vi "FipsAdjacent.vi"() -> (11 "Fips":i32[](array[numeric]))   [LabVIEW 2017] (continued)
 County, WI\"\t55119\n\"Manitowoc County, WI\"\t55071\t\"Manistee County, MI\"\t26101\n\"Manitowoc County, WI\"\t55071\t\"Mason County, MI\"\t26105\n\"Manitowoc County, WI\"\t55071\t\"Brown County, WI\"\t55009\n\"Manitowoc County, WI\"\t55071\t\"Calumet County, WI\"\t55015\n\"Manitowoc County, WI\"\t55071\t\"Kewaunee County, WI\"\t55061\n\"Manitowoc County, WI\"\t55071\t\"Manitowoc County, WI\"\t55071\n\"Manitowoc County, WI\"\t55071\t\"Sheboygan County, WI\"\t55117\n\"Marathon County, WI\"\t55073\t\"Clark County, WI\"\t55019\n\"Marathon County, WI\"\t55073\t\"Langlade County, WI\"\t55067\n\"Marathon County, WI\"\t55073\t\"Lincoln County, WI\"\t55069\n\"Marathon County, WI\"\t55073\t\"Marathon County, WI\"\t55073\n\"Marathon County, WI\"\t55073\t\"Portage County, WI\"\t55097\n\"Marathon County, WI\"\t55073\t\"Shawano County, WI\"\t55115\n\"Marathon County, WI\"\t55073\t\"Taylor County, WI\"\t55119\n\"Marathon County, WI\"\t55073\t\"Waupaca County, WI\"\t55135\n\"Marathon County, WI\"\t55073\t\"Wood County, WI\"\t55141\n\"Marinette County, WI\"\t55075\t\"Dickinson County, MI\"\t26043\n\"Marinette County, WI\"\t55075\t\"Menominee County, MI\"\t26109\n\"Marinette County, WI\"\t55075\t\"Door County, WI\"\t55029\n\"Marinette County, WI\"\t55075\t\"Florence County, WI\"\t55037\n\"Marinette County, WI\"\t55075\t\"Forest County, WI\"\t55041\n\"Marinette County, WI\"\t55075\t\"Marinette County, WI\"\t55075\n\"Marinette County, WI\"\t55075\t\"Oconto County, WI\"\t55083\n\"Marquette County, WI\"\t55077\t\"Adams County, WI\"\t55001\n\"Marquette County, WI\"\t55077\t\"Columbia County, WI\"\t55021\n\"Marquette County, WI\"\t55077\t\"Green Lake County, WI\"\t55047\n\"Marquette County, WI\"\t55077\t\"Marquette County, WI\"\t55077\n\"Marquette County, WI\"\t55077\t\"Waushara County, WI\"\t55137\n\"Menominee County, WI\"\t55078\t\"Langlade County, WI\"\t55067\n\"Menominee County, WI\"\t55078\t\"Menominee County, WI\"\t55078\n\"Menominee County, WI\"\t55078\t\"Oconto County, WI\"\t55083\n\"Menominee County, WI\"\t55078\t\"Shawano County, WI\"\t55115\n\"Milwaukee County, WI\"\t55079\t\"Muskegon County, MI\"\t26121\n\"Milwaukee County, WI\"\t55079\t\"Ottawa County, MI\"\t26139\n\"Milwaukee County, WI\"\t55079\t\"Milwaukee County, WI\"\t55079\n\"Milwaukee County, WI\"\t55079\t\"Ozaukee County, WI\"\t55089\n\"Milwaukee County, WI\"\t55079\t\"Racine County, WI\"\t55101\n\"Milwaukee County, WI\"\t55079\t\"Washington County, WI\"\t55131\n\"Milwaukee County, WI\"\t55079\t\"Waukesha County, WI\"\t55133\n\"Monroe County, WI\"\t55081\t\"Jackson County, WI\"\t55053\n\"Monroe County, WI\"\t55081\t\"Juneau County, WI\"\t55057\n\"Monroe County, WI\"\t55081\t\"La Crosse County, WI\"\t55063\n\"Monroe County, WI\"\t55081\t\"Monroe County, WI\"\t55081\n\"Monroe County, WI\"\t55081\t\"Vernon County, WI\"\t55123\n\"Oconto County, WI\"\t55083\t\"Brown County, WI\"\t55009\n\"Oconto County, WI\"\t55083\t\"Door County, WI\"\t55029\n\"Oconto County, WI\"\t55083\t\"Forest County, WI\"\t55041\n\"Oconto County, WI\"\t55083\t\"Langlade County, WI\"\t55067\n\"Oconto County, WI\"\t55083\t\"Marinette County, WI\"\t55075\n\"Oconto County, WI\"\t55083\t\"Menominee County, WI\"\t55078\n\"Oconto County, WI\"\t55083\t\"Oconto County, WI\"\t55083\n\"Oconto County, WI\"\t55083\t\"Shawano County, WI\"\t55115\n\"Oneida County, WI\"\t55085\t\"Forest County, WI\"\t55041\n\"Oneida County, WI\"\t55085\t\"Langlade County, WI\"\t55067\n\"Oneida County, WI\"\t55085\t\"Lincoln County, WI\"\t55069\n\"Oneida County, WI\"\t55085\t\"Oneida County, WI\"\t55085\n\"Oneida County, WI\"\t55085\t\"Price County, WI\"\t55099\n\"Oneida County, WI\"\t55085\t\"Vilas County, WI\"\t55125\n\"Outagamie County, WI\"\t55087\t\"Brown County, WI\"\t55009\n\"Outagamie County, WI\"\t55087\t\"Calumet County, WI\"\t55015\n\"Outagamie County, WI\"\t55087\t\"Outagamie County, WI\"\t55087\n\"Outagamie County, WI\"\t55087\t\"Shawano County, WI\"\t55115\n\"Outagamie County, WI\"\t55087\t\"Waupaca County, WI\"\t55135\n\"Outagamie County, WI\"\t55087\t\"Winnebago County, WI\"\t55139\n\"Ozaukee County, WI\"\t55089\t\"Muskegon County, MI\"\t26121\n\"Ozaukee County, WI\"\t55089\t\"Oceana County, MI\"\t26127\n\"Ozaukee County, WI\"\t55089\t\"Milwaukee County, WI\"\t55079\n\"Ozaukee County, WI\"\t55089\t\"Ozaukee County, WI\"\t55089\n\"Ozaukee County, WI\"\t55089\t\"Sheboygan County, WI\"\t55117\n\"Ozaukee County, WI\"\t55089\t\"Washington County, WI\"\t55131\n\"Ozaukee County, WI\"\t55089\t\"Waukesha County, WI\"\t55133\n\"Pepin County, WI\"\t55091\t\"Goodhue County, MN\"\t27049\n\"Pepin County, WI\"\t55091\t\"Wabasha County, MN\"\t27157\n\"Pepin County, WI\"\t55091\t\"Buffalo County, WI\"\t55011\n\"Pepin County, WI\"\t55091\t\"Dunn County, WI\"\t55033\n\"Pepin County, WI\"\t55091\t\"Eau Claire County, WI\"\t55035\n\"Pepin County, WI\"\t55091\t\"Pepin County, WI\"\t55091\n\"Pepin County, WI\"\t55091\t\"Pierce County, WI\"\t55093\n\"Pierce County, WI\"\t55093\t\"Dakota County, MN\"\t27037\n\"Pierce County, WI\"\t55093\t\"Goodhue County, MN\"\t27049\n\"Pierce County, WI\"\t55093\t\"Washington County, MN\"\t27163\n\"Pierce County, WI\"\t55093\t\"Dunn County, WI\"\t55033\n\"Pierce County, WI\"\t55093\t\"Pepin County, WI\"\t55091\n\"Pierce County, WI\"\t55093\t\"Pierce County, WI\"\t55093\n\"Pierce County, WI\"\t55093\t\"St. Croix County, WI\"\t55109\n\"Polk County, WI\"\t55095\t\"Chisago County, MN\"\t27025\n\"Polk County, WI\"\t55095\t\"Washington County, MN\"\t27163\n\"Polk County, WI\"\t55095\t\"Barron County, WI\"\t55005\n\"Polk County, WI\"\t55095\t\"Burnett County, WI\"\t55013\n\"Polk County, WI\"\t55095\t\"Dunn County, WI\"\t55033\n\"Polk County, WI\"\t55095\t\"Polk County, WI\"\t55095\n\"Polk County, WI\"\t55095\t\"St. Croix County, WI\"\t55109\n\"Portage County, WI\"\t55097\t\"Adams County, WI\"\t55001\n\"Portage County, WI\"\t55097\t\"Marathon County, WI\"\t55073\n\"Portage County, WI\"\t55097\t\"Portage County, WI\"\t55097\n\"Portage County, WI\"\t55097\t\"Shawano County, WI\"\t55115\n\"Portage County, WI\"\t55097\t\"Waupaca County, WI\"\t55135\n\"Portage County, WI\"\t55097\t\"Waushara County, WI\"\t55137\n\"Portage County, WI\"\t55097\t\"Wood County, WI\"\t55141\n\"Price County, WI\"\t55099\t\"Ashland County, WI\"\t55003\n\"Price County, WI\"\t55099\t\"Iron County, WI\"\t55051\n\"Price County, WI\"\t55099\t\"Lincoln County, WI\"\t55069\n\"Price County, WI\"\t55099\t\"Oneida County, WI\"\t55085\n\"Price County, WI\"\t55099\t\"Price County, WI\"\t55099\n\"Price County, WI\"\t55099\t\"Rusk County, WI\"\t55107\n\"Price County, WI\"\t55099\t\"Sawyer County, WI\"\t55113\n\"Price County, WI\"\t55099\t\"Taylor County, WI\"\t55119\n\"Price County, WI\"\t55099\t\"Vilas County, WI\"\t55125\n\"Racine County, WI\"\t55101\t\"Allegan County, MI\"\t26005\n\"Racine County, WI\"\t55101\t\"Ottawa County, MI\"\t26139\n\"Racine County, WI\"\t55101\t\"Kenosha County, WI\"\t55059\n\"Racine County, WI\"\t55101\t\"Milwaukee County, WI\"\t55079\n\"Racine County, WI\"\t55101\t\"Racine County, WI\"\t55101\n\"Racine County, WI\"\t55101\t\"Walworth County, WI\"\t55127\n\"Racine County, WI\"\t55101\t\"Waukesha County, WI\"\t55133\n\"Richland County, WI\"\t55103\t\"Crawford County, WI\"\t55023\n\"Richland County, WI\"\t55103\t\"Grant County, WI\"\t55043\n\"Richland County, WI\"\t55103\t\"Iowa County, WI\"\t55049\n\"Richland County, WI\"\t55103\t\"Richland County, WI\"\t55103\n\"Richland County, WI\"\t55103\t\"Sauk County, WI\"\t55111\n\"Richland County, WI\"\t55103\t\"Vernon County, WI\"\t55123\n\"Rock County, WI\"\t55105\t\"Boone County, IL\"\t17007\n\"Rock County, WI\"\t55105\t\"Winnebago County, IL\"\t17201\n\"Rock County, WI\"\t55105\t\"Dane County, WI\"\t55025\n\"Rock County, WI\"\t55105\t\"Green County, WI\"\t55045\n\"Rock County, WI\"\t55105\t\"Jefferson County, WI\"\t55055\n\"Rock County, WI\"\t55105\t\"Rock County, WI\"\t55105\n\"Rock County, WI\"\t55105\t\"Walworth County, WI\"\t55127\n\"Rusk County, WI\"\t55107\t\"Barron County, WI\"\t55005\n\"Rusk County, WI\"\t55107\t\"Chippewa County, WI\"\t55017\n\"Rusk County, WI\"\t55107\t\"Price County, WI\"\t55099\n\"Rusk County, WI\"\t55107\t\"Rusk County, WI\"\t55107\n\"Rusk County, WI\"\t55107\t\"Sawyer County, WI\"\t55113\n\"Rusk County, WI\"\t55107\t\"Taylor County, WI\"\t55119\n\"Rusk County, WI\"\t55107\t\"Washburn County, WI\"\t55129\n\"St. Croix County, WI\"\t55109\t\"Washington County, MN\"\t27163\n\"St. Croix County, WI\"\t55109\t\"Barron County, WI\"\t55005\n\"St. Croix County, WI\"\t55109\t\"Dunn County, WI\"\t55033\n\"St. Croix County, WI\"\t55109\t\"Pierce County, WI\"\t55093\n\"St. Croix County, WI\"\t55109\t\"Polk County, WI\"\t55095\n\"St. Croix County, WI\"\t55109\t\"St. Croix County, WI\"\t55109\n\"Sauk County, WI\"\t55111\t\"Adams County, WI\"\t55001\n\"Sauk County, WI\"\t55111\t\"Columbia County, WI\"\t55021\n\"Sauk County, WI\"\t55111\t\"Dane County, WI\"\t55025\n\"Sauk County, WI\"\t55111\t\"Iowa County, WI\"\t55049\n\"Sauk County, WI\"\t55111\t\"Juneau County, WI\"\t55057\n\"Sauk County, WI\"\t55111\t\"Richland County, WI\"\t55103\n\"Sauk County, WI\"\t55111\t\"Sauk County, WI\"\t55111\n\"Sauk County, WI\"\t55111\t\"Vernon County, WI\"\t55123\n\"Sawyer County, WI\"\t55113\t\"Ashland County, WI\"\t55003\n\"Sawyer County, WI\"\t55113\t\"Barron County, WI\"\t55005\n\"Sawyer County, WI\"\t55113\t\"Bayfield County, WI\"\t55007\n\"Sawyer County, WI\"\t55113\t\"Douglas County, WI\"\t55031\n\"Sawyer County, WI\"\t55113\t\"Price County, WI\"\t55099\n\"Sawyer County, WI\"\t55113\t\"Rusk County, WI\"\t55107\n\"Sawyer County, WI\"\t55113\t\"Sawyer County, WI\"\t55113\n\"Sawyer County, WI\"\t55113\t\"Washburn County, WI\"\t55129\n\"Shawano County, WI\"\t55115\t\"Brown County, WI\"\t55009\n\"Shawano County, WI\"\t55115\t\"Langlade County, WI\"\t55067\n\"Shawano County, WI\"\t55115\t\"Marathon County, WI\"\t55073\n\"Shawano County, WI\"\t55115\t\"Menominee County, WI\"\t55078\n\"Shawano County, WI\"\t55115\t\"Oconto County, WI\"\t55083\n\"Shawano County, WI\"\t55115\t\"Outagamie County, WI\"\t55087\n\"Shawano County, WI\"\t55115\t\"Portage County, WI\"\t55097\n\"Shawano County, WI\"\t55115\t\"Shawano County, WI\"\t55115\n\"Shawano County, WI\"\t55115\t\"Waupaca County, WI\"\t55135\n\"Sheboygan County, WI\"\t55117\t\"Mason County, MI\"\t26105\n\"Sheboygan County, WI\"\t55117\t\"Oceana County, MI\"\t26127\n\"Sheboygan County, WI\"\t55117\t\"Calumet County, WI\"\t55015\n\"Sheboygan County, WI\"\t55117\t\"Fond du Lac County, WI\"\t55039\n\"Sheboygan County, WI\"\t55117\t\"Manitowoc County, WI\"\t55071\n\"Sheboygan County, WI\"\t55117\t\"Ozaukee County, WI\"\t55089\n\"Sheboygan County, WI\"\t55117\t\"Sheboygan County, WI\"\t55117\n\"Sheboygan County, WI\"\t55117\t\"Washington County, WI\"\t55131\n\"Taylor County, WI\"\t55119\t\"Chippewa County, WI\"\t55017\n\"Taylor County, WI\"\t55119\t\"Clark County, WI\"\t55019\n\"Taylor County, WI\"\t55119\t\"Lincoln County, WI\"\t55069\n\"Taylor County, WI\"\t55119\t\"Marathon County, WI\"\t55073\n\"Taylor County, WI\"\t55119\t\"Price County, WI\"\t55099\n\"Taylor County, WI\"\t55119\t\"Rusk County, WI\"\t55107\n\"Taylor County, WI\"\t55119\t\"Taylor County, WI\"\t55119\n\"Trempealeau County, WI\"\t55121\t\"Winona County, MN\"\t27169\n\"Trempealeau County, WI\"\t55121\t\"Buffalo County, WI\"\t55011\n\"Trempealeau County, WI\"\t55121\t\"Eau Claire County, WI\"\t55035\n\"Trempealeau County, WI\"\t55121\t\"Jackson County, WI\"\t55053\n\"Trempealeau County, WI\"\t55121\t\"La Crosse County, WI\"\t55063\n\"Trempealeau County, WI\"\t55121\t\"Trempealeau County, WI\"\t55121\n\"Vernon County, WI\"\t55123\t\"Allamakee County, IA\"\t19005\n\"Vernon County, WI\"\t55123\t\"Houston County, MN\"\t27055\n\"Vernon County, WI\"\t55123\t\"Crawford County, WI\"\t55023\n\"Vernon County, WI\"\t55123\t\"Juneau County, WI\"\t55057\n\"Vernon County, WI\"\t55123\t\"La Crosse County, WI\"\t55063\n\"Vernon County, WI\"\t55123\t\"Monroe County, WI\"\t55081\n\"Vernon County, WI\"\t55123\t\"Richland County, WI\"\t55103\n\"Vernon County, WI\"\t55123\t\"Sauk County, WI\"\t55111\n\"Vernon County, WI\"\t55123\t\"Vernon County, WI\"\t55123\n\"Vilas County, WI\"\t55125\t\"Gogebic County, MI\"\t26053\n\"Vilas County, WI\"\t55125\t\"Iron County, MI\"\t26071\n\"Vilas County, WI\"\t55125\t\"Forest County, WI\"\t55041\n\"Vilas County, WI\"\t55125\t\"Iron County, WI\"\t55051\n\"Vilas County, WI\"\t55125\t\"Oneida County, WI\"\t55085\n\"Vilas County, WI\"\t55125\t\"Price County, WI\"\t55099\n\"Vilas County, WI\"\t55125\t\"Vilas County, WI\"\t55125\n\"Walworth County, WI\"\t55127\t\"Boone County, IL\"\t17007\n\"Walworth County, WI\"\t55127\t\"McHenry County, IL\"\t17111\n\"Walworth County, WI\"\t55127\t\"Jefferson County, WI\"\t55055\n\"Walworth County, WI\"\t55127\t\"Kenosha County, WI\"\t55059\n\"Walworth County, WI\"\t55127\t\"Racine County, WI\"\t55101\n\"Walworth County, WI\"\t55127\t\"Rock County, WI\"\t55105\n\"Walworth County, WI\"\t55127\t\"Walworth County, WI\"\t55127\n\"Walworth County, WI\"\t55127\t\"Waukesha County, WI\"\t55133\n\"Washburn County, WI\"\t55129\t\"Barron County, WI\"\t55005\n\"Washburn County, WI\"\t55129\t\"Bayfield County, WI\"\t55007\n\"Washburn County, WI\"\t55129\t\"Burnett County, WI\"\t55013\n\"Washburn County, WI\"\t55129\t\"Douglas County, WI\"\t55031\n\"Washburn County, WI\"\t55129\t\"Rusk County, WI\"\t55107\n\"Washburn County, WI\"\t55129\t\"Sawyer County, WI\"\t55113\n\"Washburn County, WI\"\t55129\t\"Washburn County, WI\"\t55129\n\"Washington County, WI\"\t55131\t\"Dodge County, WI\"\t55027\n\"Washington County, WI\"\t55131\t\"Fond du Lac County, WI\"\t55039\n\"Washington County, WI\"\t55131\t\"Milwaukee County, WI\"\t55079\n\"Washington County, WI\"\t55131\t\"Ozaukee County, WI\"\t55089\n\"Washington County, WI\"\t55131\t\"Sheboygan County, WI\"\t55117\n\"Washington County, WI\"\t55131\t\"Washington County, WI\"\t55131\n\"Washington County, WI\"\t55131\t\"Waukesha County, WI\"\t55133\n\"Waukesha County, WI\"\t55133\t\"Dodge County, WI\"\t55027\n\"Waukesha County, WI\"\t55133\t\"Jefferson County, WI\"\t55055\n\"Waukesha County, WI\"\t55133\t\"Milwaukee County, WI\"\t55079\n\"Waukesha County, WI\"\t55133\t\"Ozaukee County, WI\"\t55089\n\"Waukesha County, WI\"\t55133\t\"Racine County, WI\"\t55101\n\"Waukesha County, WI\"\t55133\t\"Walworth County, WI\"\t55127\n\"Waukesha County, WI\"\t55133\t\"Washington County, WI\"\t55131\n\"Waukesha County, WI\"\t55133\t\"Waukesha County, WI\"\t55133\n\"Waupaca County, WI\"\t55135\t\"Marathon County, WI\"\t55073\n\"Waupaca County, WI\"\t55135\t\"Outagamie County, WI\"\t55087\n\"Waupaca County, WI\"\t55135\t\"Portage County, WI\"\t55097\n\"Waupaca County, WI\"\t55135\t\"Shawano County, WI\"\t55115\n\"Waupaca County, WI\"\t55135\t\"Waupaca County, WI\"\t55135\n\"Waupaca County, WI\"\t55135\t\"Waushara County, WI\"\t55137\n\"Waupaca County, WI\"\t55135\t\"Winnebago County, WI\"\t55139\n\"Waushara County, WI\"\t55137\t\"Adams County, WI\"\t55001\n\"Waushara County, WI\"\t55137\t\"Green Lake County, WI\"\t55047\n\"Waushara County, WI\"\t55137\t\"Marquette County, WI\"\t55077\n\"Waushara County, WI\"\t55137\t\"Portage County, WI\"\t55097\n\"Waushara County, WI\"\t55137\t\"Waupaca County, WI\"\t55135\n\"Waushara County, WI\"\t55137\t\"Waushara County, WI\"\t55137\n\"Waushara County, WI\"\t55137\t\"Winnebago County, WI\"\t55139\n\"Winnebago County, WI\"\t55139\t\"Calumet County, WI\"\t55015\n\"Winnebago County, WI\"\t55139\t\"Fond du Lac County, WI\"\t55039\n\"Winnebago County, WI\"\t55139\t\"Green Lake County, WI\"\t55047\n\"Winnebago County, WI\"\t55139\t\"Outagamie County, WI\"\t55087\n\"Winnebago County, WI\"\t55139\t\"Waupaca County, WI\"\t55135\n\"Winnebago County, WI\"\t55139\t\"Waushara County, WI\"\t55137\n\"Winnebago County, WI\"\t55139\t\"Winnebago County, WI\"\t55139\n\"Wood County, WI\"\t55141\t\"Adams County, WI\"\t55001\n\"Wood County, WI\"\t55141\t\"Clark County, WI\"\t55019\n\"Wood County, WI\"\t55141\t\"Jackson County, WI\"\t55053\n\"Wood County, WI\"\t55141\t\"Juneau County, WI\"\t55057\n\"Wood County, WI\"\t55141\t\"Marathon County, WI\"\t55073\n\"Wood County, WI\"\t55141\t\"Portage County, WI\"\t55097\n\"Wood County, WI\"\t55141\t\"Wood County, WI\"\t55141\n\"Albany County, WY\"\t56001\t\"Jackson County, CO\"\t08057\n\"Albany County, WY\"\t56001\t\"Larimer County, CO\"\t08069\n\"Albany County, WY\"\t56001\t\"Albany County, WY\"\t56001\n\"Albany County, WY\"\t56001\t\"Carbon County, WY\"\t56007\n\"Albany County, WY\"\t56001\t\"Converse County, WY\"\t56009\n\"Albany County, WY\"\t56001\t\"Laramie County, WY\"\t56021\n\"Albany County, WY\"\t56001\t\"Platte County, WY\"\t56031\n\"Big Horn County, WY\"\t56003\t\"Big Horn County, MT\"\t30003\n\"Big Horn County, WY\"\t56003\t\"Carbon County, MT\"\t30009\n\"Big Horn County, WY\"\t56003\t\"Big Horn County, WY\"\t56003\n\"Big Horn County, WY\"\t56003\t\"Johnson County, WY\"\t56019\n\"Big Horn County, WY\"\t56003\t\"Park County, WY\"\t56029\n\"Big Horn County, WY\"\t56003\t\"Sheridan County, WY\"\t56033\n\"Big Horn County, WY\"\t56003\t\"Washakie County, WY\"\t56043\n\"Campbell County, WY\"\t56005\t\"Powder River County, MT\"\t30075\n\"Campbell County, WY\"\t56005\t\"Campbell County, WY\"\t56005\n\"Campbell County, WY\"\t56005\t\"Converse County, WY\"\t56009\n\"Campbell County, WY\"\t56005\t\"Crook County, WY\"\t56011\n\"Campbell County, WY\"\t56005\t\"Johnson County, WY\"\t56019\n\"Campbell County, WY\"\t56005\t\"Sheridan County, WY\"\t56033\n\"Campbell County, WY\"\t56005\t\"Weston County, WY\"\t56045\n\"Carbon County, WY\"\t56007\t\"Jackson County, CO\"\t08057\n\"Carbon County, WY\"\t56007\t\"Moffat County, CO\"\t08081\n\"Carbon County, WY\"\t56007\t\"Routt County, CO\"\t08107\n\"Carbon County, WY\"\t56007\t\"Albany County, WY\"\t56001\n\"Carbon County, WY\"\t56007\t\"Carbon County, WY\"\t56007\n\"Carbon County, WY\"\t56007\t\"Converse County, WY\"\t56009\n\"Carbon County, WY\"\t56007\t\"Fremont County, WY\"\t56013\n\"Carbon County, WY\"\t56007\t\"Natrona County, WY\"\t56025\n\"Carbon County, WY\"\t56007\t\"Sweetwater County, WY\"\t56037\n\"Converse County, WY\"\t56009\t\"Albany County, WY\"\t56001\n\"Converse County, WY\"\t56009\t\"Campbell County, WY\"\t56005\n\"Converse County, WY\"\t56009\t\"Carbon County, WY\"\t56007\n\"Converse County, WY\"\t56009\t\"Converse County, WY\"\t56009\n\"Converse County, WY\"\t56009\t\"Johnson County, WY\"\t56019\n\"Converse County, WY\"\t56009\t\"Natrona County, WY\"\t56025\n\"Converse County, WY\"\t56009\t\"Niobrara County, WY\"\t56027\n\"Converse County, WY\"\t56009\t\"Platte County, WY\"\t56031\n\"Converse County, WY\"\t56009\t\"Weston County, WY\"\t56045\n\"Crook County, WY\"\t56011\t\"Carter County, MT\"\t30011\n\"Crook County, WY\"\t56011\t\"Powder River County, MT\"\t30075\n\"Crook County, WY\"\t56011\t\"Butte County, SD\"\t46019\n\"Crook County, WY\"\t56011\t\"Lawrence County, SD\"\t46081\n\"Crook County, WY\"\t56011\t\"Campbell County, WY\"\t56005\n\"Crook County, WY\"\t56011\t\"Crook County, WY\"\t56011\n\"Crook County, WY\"\t56011\t\"Weston County, WY\"\t56045\n\"Fremont County, WY\"\t56013\t\"Carbon County, WY\"\t56007\n\"Fremont County, WY\"\t56013\t\"Fremont County, WY\"\t56013\n\"Fremont County, WY\"\t56013\t\"Hot Springs County, WY\"\t56017\n\"Fremont County, WY\"\t56013\t\"Natrona County, WY\"\t56025\n\"Fremont County, WY\"\t56013\t\"Park County, WY\"\t56029\n\"Fremont County, WY\"\t56013\t\"Sublette County, WY\"\t56035\n\"Fremont County, WY\"\t56013\t\"Sweetwater County, WY\"\t56037\n\"Fremont County, WY\"\t56013\t\"Teton County, WY\"\t56039\n\"Fremont County, WY\"\t56013\t\"Washakie County, WY\"\t56043\n\"Goshen County, WY\"\t56015\t\"Banner County, NE\"\t31007\n\"Goshen County, WY\"\t56015\t\"Scotts Bluff County, NE\"\t31157\n\"Goshen County, WY\"\t56015\t\"Sioux County, NE\"\t31165\n\"Goshen County, WY\"\t56015\t\"Goshen County, WY\"\t56015\n\"Goshen County, WY\"\t56015\t\"Laramie County, WY\"\t56021\n\"Goshen County, WY\"\t56015\t\"Niobrara County, WY\"\t56027\n\"Goshen County, WY\"\t56015\t\"Platte County, WY\"\t56031\n\"Hot Springs County, WY\"\t56017\t\"Fremont County, WY\"\t56013\n\"Hot Springs County, WY\"\t56017\t\"Hot Springs County, WY\"\t56017\n\"Hot Springs County, WY\"\t56017\t\"Park County, WY\"\t56029\n\"Hot Springs County, WY\"\t56017\t\"Washakie County, WY\"\t56043\n\"Johnson County, WY\"\t56019\t\"Big Horn County, WY\"\t56003\n\"Johnson County, WY\"\t56019\t\"Campbell County, WY\"\t56005\n\"Johnson County, WY\"\t56019\t\"Converse County, WY\"\t56009\n\"Johnson County, WY\"\t56019\t\"Johnson County, WY\"\t56019\n\"Johnson County, WY\"\t56019\t\"Natrona County, WY\"\t56025\n\"Johnson County, WY\"\t56019\t\"Sheridan County, WY\"\t56033\n\"Johnson County, WY\"\t56019\t\"Washakie County, WY\"\t56043\n\"Laramie County, WY\"\t56021\t\"Larimer County, CO\"\t08069\n\"Laramie County, WY\"\t56021\t\"Weld County, CO\"\t08123\n\"Laramie County, WY\"\t56021\t\"Banner County, NE\"\t31007\n\"Laramie County, WY\"\t56021\t\"Kimball County, NE\"\t31105\n\"Laramie County, WY\"\t56021\t\"Albany County, WY\"\t56001\n\"Laramie County, WY\"\t56021\t\"Goshen County, WY\"\t56015\n\"Laramie County, WY\"\t56021\t\"Laramie County, WY\"\t56021\n\"Laramie County, WY\"\t56021\t\"Platte County, WY\"\t56031\n\"Lincoln County, WY\"\t56023\t\"Bear Lake County, ID\"\t16007\n\"Lincoln County, WY\"\t56023\t\"Bonneville County, ID\"\t16019\n\"Lincoln County, WY\"\t56023\t\"Caribou County, ID\"\t16029\n\"Lincoln County, WY\"\t56023\t\"Rich County, UT\"\t49033\n\"Lincoln County, WY\"\t56023\t\"Lincoln County, WY\"\t56023\n\"Lincoln County, WY\"\t56023\t\"Sublette County, WY\"\t56035\n\"Lincoln County, WY\"\t56023\t\"Sweetwater County, WY\"\t56037\n\"Lincoln County, WY\"\t56023\t\"Teton County, WY\"\t56039\n\"Lincoln County, WY\"\t56023\t\"Uinta County, WY\"\t56041\n\"Natrona County, WY\"\t56025\t\"Carbon County, WY\"\t56007\n\"Natrona County, WY\"\t56025\t\"Converse County, WY\"\t56009\n\"Natrona County, WY\"\t56025\t\"Fremont County, WY\"\t56013\n\"Natrona County, WY\"\t56025\t\"Johnson County, WY\"\t56019\n\"Natrona County, WY\"\t56025\t\"Natrona County, WY\"\t56025\n\"Natrona County, WY\"\t56025\t\"Washakie County, WY\"\t56043\n\"Niobrara County, WY\"\t56027\t\"Sioux County, NE\"\t31165\n\"Niobrara County, WY\"\t56027\t\"Custer County, SD\"\t46033\n\"Niobrara County, WY\"\t56027\t\"Fall River County, SD\"\t46047\n\"Niobrara County, WY\"\t56027\t\"Converse County, WY\"\t56009\n\"Niobrara County, WY\"\t56027\t\"Goshen County, WY\"\t56015\n\"Niobrara County, WY\"\t56027\t\"Niobrara County, WY\"\t56027\n\"Niobrara County, WY\"\t56027\t\"Platte County, WY\"\t56031\n\"Niobrara County, WY\"\t56027\t\"Weston County, WY\"\t56045\n\"Park County, WY\"\t56029\t\"Carbon County, MT\"\t30009\n\"Park County, WY\"\t56029\t\"Gallatin County, MT\"\t30031\n\"Park County, WY\"\t56029\t\"Park County, MT\"\t30067\n\"Park County, WY\"\t56029\t\"Big Horn County, WY\"\t56003\n\"Park County, WY\"\t56029\t\"Fremont County, WY\"\t56013\n\"Park County, WY\"\t56029\t\"Hot Springs County, WY\"\t56017\n\"Park County, WY\"\t56029\t\"Park County, WY\"\t56029\n\"Park County, WY\"\t56029\t\"Teton County, WY\"\t56039\n\"Park County, WY\"\t56029\t\"Washakie County, WY\"\t56043\n\"Platte County, WY\"\t56031\t\"Albany County, WY\"\t56001\n\"Platte County, WY\"\t56031\t\"Converse County, WY\"\t56009\n\"Platte County, WY\"\t56031\t\"Goshen County, WY\"\t56015\n\"Platte County, WY\"\t56031\t\"Laramie County, WY\"\t56021\n\"Platte County, WY\"\t56031\t\"Niobrara County, WY\"\t56027\n\"Platte County, WY\"\t56031\t\"Platte County, WY\"\t56031\n\"Sheridan County, WY\"\t56033\t\"Big Horn County, MT\"\t30003\n\"Sheridan County, WY\"\t56033\t\"Powder River County, MT\"\t30075\n\"Sheridan County, WY\"\t56033\t\"Big Horn County, WY\"\t56003\n\"Sheridan County, WY\"\t56033\t\"Campbell County, WY\"\t56005\n\"Sheridan County, WY\"\t56033\t\"Johnson County, WY\"\t56019\n\"Sheridan County, WY\"\t56033\t\"Sheridan County, WY\"\t56033\n\"Sublette County, WY\"\t56035\t\"Fremont County, WY\"\t56013\n\"Sublette County, WY\"\t56035\t\"Lincoln County, WY\"\t56023\n\"Sublette County, WY\"\t56035\t\"Sublette County, WY\"\t56035\n\"Sublette County, WY\"\t56035\t\"Sweetwater County, WY\"\t56037\n\"Sublette County, WY\"\t56035\t\"Teton County, WY\"\t56039\n\"Sweetwater County, WY\"\t56037\t\"Moffat County, CO\"\t08081\n\"Sweetwater County, WY\"\t56037\t\"Daggett County, UT\"\t49009\n\"Sweetwater County, WY\"\t56037\t\"Summit County, UT\"\t49043\n\"Sweetwater County, WY\"\t56037\t\"Carbon County, WY\"\t56007\n\"Sweetwater County, WY\"\t56037\t\"Fremont County, WY\"\t56013\n\"Sweetwater County, WY\"\t56037\t\"Lincoln County, WY\"\t56023\n\"Sweetwater County, WY\"\t56037\t\"Sublette County, WY\"\t56035\n\"Sweetwater County, WY\"\t56037\t\"Sweetwater County, WY\"\t56037\n\"Sweetwater County, WY\"\t56037\t\"Uinta County, WY\"\t56041\n\"Teton County, WY\"\t56039\t\"Bonneville County, ID\"\t16019\n\"Teton County, WY\"\t56039\t\"Fremont County, ID\"\t16043\n\"Teton County, WY\"\t56039\t\"Teton County, ID\"\t16081\n\"Teton County, WY\"\t56039\t\"Gallatin County, MT\"\t30031\n\"Teton County, WY\"\t56039\t\"Fremont County, WY\"\t56013\n\"Teton County, WY\"\t56039\t\"Lincoln County, WY\"\t56023\n\"Teton County, WY\"\t56039\t\"Park County, WY\"\t56029\n\"Teton County, WY\"\t56039\t\"Sublette County, WY\"\t56035\n\"Teton County, WY\"\t56039\t\"Teton County, WY\"\t56039\n\"Uinta County, WY\"\t56041\t\"Rich County, UT\"\t49033\n\"Uinta County, WY\"\t56041\t\"Summit County, UT\"\t49043\n\"Uinta County, WY\"\t56041\t\"Lincoln County, WY\"\t56023\n\"Uinta County, WY\"\t56041\t\"Sweetwater County, WY\"\t56037\n\"Uinta County, WY\"\t56041\t\"Uinta County, WY\"\t56041\n\"Washakie County, WY\"\t56043\t\"Big Horn County, WY\"\t56003\n\"Washakie County, WY\"\t56043\t\"Fremont County, WY\"\t56013\n\"Washakie County, WY\"\t56043\t\"Hot Springs County, WY\"\t56017\n\"Washakie County, WY\"\t56043\t\"Johnson County, WY\"\t56019\n\"Washakie County, WY\"\t56043\t\"Natrona County, WY\"\t56025\n\"Washakie County, WY\"\t56043\t\"Park County, WY\"\t56029\n\"Washakie County, WY\"\t56043\t\"Washakie County, WY\"\t56043\n\"Weston County, WY\"\t56045\t\"Custer County, SD\"\t46033\n\"Weston County, WY\"\t56045\t\"Lawrence County, SD\"\t46081\n\"Weston County, WY\"\t56045\t\"Pennington County, SD\"\t46103\n\"Weston County, WY\"\t56045\t\"Campbell County, WY\"\t56005\n\"Weston County, WY\"\t56045\t\"Converse County, WY\"\t56009\n\"Weston County, WY\"\t56045\t\"Crook County, WY\"\t56011\n\"Weston County, WY\"\t56045\t\"Niobrara County, WY\"\t56027\n\"Weston County, WY\"\t56045\t\"Weston County, WY\"\t56045\n\"Adjuntas Municipio, PR\"\t72001\t\"Adjuntas Municipio, PR\"\t72001\n\"Adjuntas Municipio, PR\"\t72001\t\"Guayanilla Municipio, PR\"\t72059\n\"Adjuntas Municipio, PR\"\t72001\t\"Lares Municipio, PR\"\t72081\n\"Adjuntas Municipio, PR\"\t72001\t\"Pe?uelas Municipio, PR\"\t72111\n\"Adjuntas Municipio, PR\"\t72001\t\"Ponce Municipio, PR\"\t72113\n\"Adjuntas Municipio, PR\"\t72001\t\"Utuado Municipio, PR\"\t72141\n\"Adjuntas Municipio, PR\"\t72001\t\"Yauco Municipio, PR\"\t72153\n\"Aguada Municipio, PR\"\t72003\t\"Aguada Municipio, PR\"\t72003\n\"Aguada Municipio, PR\"\t72003\t\"Aguadilla Municipio, PR\"\t72005\n\"Aguada Municipio, PR\"\t72003\t\"A?asco Municipio, PR\"\t72011\n\"Aguada Municipio, PR\"\t72003\t\"Moca Municipio, PR\"\t72099\n\"Aguada Municipio, PR\"\t72003\t\"Rinc?n Municipio, PR\"\t72117\n\"Aguadilla Municipio, PR\"\t72005\t\"Aguada Municipio, PR\"\t72003\n\"Aguadilla Municipio, PR\"\t72005\t\"Aguadilla Municipio, PR\"\t72005\n\"Aguadilla Municipio, PR\"\t72005\t\"Isabela Municipio, PR\"\t72071\n\"Aguadilla Municipio, PR\"\t72005\t\"Moca Municipio, PR\"\t72099\n\"Aguas Buenas Municipio, PR\"\t72007\t\"Aguas Buenas Municipio, PR\"\t72007\n\"Aguas Buenas Municipio, PR\"\t72007\t\"Bayam?n Municipio, PR\"\t72021\n\"Aguas Buenas Municipio, PR\"\t72007\t\"Caguas Municipio, PR\"\t72025\n\"Aguas Buenas Municipio, PR\"\t72007\t\"Cidra Municipio, PR\"\t72041\n\"Aguas Buenas Municipio, PR\"\t72007\t\"Comer?o Municipio, PR\"\t72045\n\"Aguas Buenas Municipio, PR\"\t72007\t\"Guaynabo Municipio, PR\"\t72061\n\"Aguas Buenas Municipio, PR\"\t72007\t\"San Juan Municipio, PR\"\t72127\n\"Aibonito Municipio, PR\"\t72009\t\"Aibonito Municipio, PR\"\t72009\n\"Aibonito Municipio, PR\"\t72009\t\"Barranquitas Municipio, PR\"\t72019\n\"Aibonito Municipio, PR\"\t72009\t\"Cayey Municipio, PR\"\t72035\n\"Aibonito Municipio, PR\"\t72009\t\"Cidra Municipio, PR\"\t72041\n\"Aibonito Municipio, PR\"\t72009\t\"Coamo Municipio, PR\"\t72043\n\"Aibonito Municipio, PR\"\t72009\t\"Salinas Municipio, PR\"\t72123\n\"A?asco Municipio, PR\"\t72011\t\"Aguada Municipio, PR\"\t72003\n\"A?asco Municipio, PR\"\t72011\t\"A?asco Municipio, PR\"\t72011\n\"A?asco Municipio, PR\"\t72011\t\"Las Mar?as Municipio, PR\"\t72083\n\"A?asco Municipio, PR\"\t72011\t\"Mayag?ez Municipio, PR\"\t72097\n\"A?asco Municipio, PR\"\t72011\t\"Moca Municipio, PR\"\t72099\n\"A?asco Municipio, PR\"\t72011\t\"Rinc?n Municipio, PR\"\t72117\n\"A?asco Municipio, PR\"\t72011\t\"San Sebasti?n Municipio, PR\"\t72131\n\"Arecibo Municipio, PR\"\t72013\t\"Arecibo Municipio, PR\"\t72013\n\"Arecibo Municipio, PR\"\t72013\t\"Barceloneta Municipio, PR\"\t72017\n\"Arecibo Municipio, PR\"\t72013\t\"Ciales Municipio, PR\"\t72039\n\"Arecibo Municipio, PR\"\t72013\t\"Florida Municipio, PR\"\t72054\n\"Arecibo Municipio, PR\"\t72013\t\"Hatillo Municipio, PR\"\t72065\n\"Arecibo Municipio, PR\"\t72013\t\"Utuado Municipio, PR\"\t72141\n\"Arroyo Municipio, PR\"\t72015\t\"Arroyo Municipio, PR\"\t72015\n\"Arroyo Municipio, PR\"\t72015\t\"Guayama Municipio, PR\"\t72057\n\"Arroyo Municipio, PR\"\t72015\t\"Patillas Municipio, PR\"\t72109\n\"Barceloneta Municipio, PR\"\t72017\t\"Arecibo Municipio, PR\"\t72013\n\"Barceloneta Municipio, PR\"\t72017\t\"Barceloneta Municipio, PR\"\t72017\n\"Barceloneta Municipio, PR\"\t72017\t\"Florida Municipio, PR\"\t72054\n\"Barceloneta Municipio, PR\"\t72017\t\"Manat? Municipio, PR\"\t72091\n\"Barranquitas Municipio, PR\"\t72019\t\"Aibonito Municipio, PR\"\t72009\n\"Barranquitas Municipio, PR\"\t72019\t\"Barranquitas Municipio, PR\"\t72019\n\"Barranquitas Municipio, PR\"\t72019\t\"Cidra Municipio, PR\"\t72041\n\"Barranquitas Municipio, PR\"\t72019\t\"Coamo Municipio, PR\"\t72043\n\"Barranquitas Municipio, PR\"\t72019\t\"Comer?o Municipio, PR\"\t72045\n\"Barranquitas Municipio, PR\"\t72019\t\"Corozal Municipio, PR\"\t72047\n\"Barranquitas Municipio, PR\"\t72019\t\"Naranjito Municipio, PR\"\t72105\n\"Barranquitas Municipio, PR\"\t72019\t\"Orocovis Municipio, PR\"\t72107\n\"Bayam?n Municipio, PR\"\t72021\t\"Aguas Buenas Municipio, PR\"\t72007\n\"Bayam?n Municipio, PR\"\t72021\t\"Bayam?n Municipio, PR\"\t72021\n\"Bayam?n Municipio, PR\"\t72021\t\"Cata?o Municipio, PR\"\t72033\n\"Bayam?n Municipio, PR\"\t72021\t\"Comer?o Municipio, PR\"\t72045\n\"Bayam?n Municipio, PR\"\t72021\t\"Guaynabo Municipio, PR\"\t72061\n\"Bayam?n Municipio, PR\"\t72021\t\"Naranjito Municipio, PR\"\t72105\n\"Bayam?n Municipio, PR\"\t72021\t\"Toa Alta Municipio, PR\"\t72135\n\"Bayam?n Municipio, PR\"\t72021\t\"Toa Baja Municipio, PR\"\t72137\n\"Cabo Rojo Municipio, PR\"\t72023\t\"Cabo Rojo Municipio, PR\"\t72023\n\"Cabo Rojo Municipio, PR\"\t72023\t\"Hormigueros Municipio, PR\"\t72067\n\"Cabo Rojo Municipio, PR\"\t72023\t\"Lajas Municipio, PR\"\t72079\n\"Cabo Rojo Municipio, PR\"\t72023\t\"Mayag?ez Municipio, PR\"\t72097\n\"Cabo Rojo Municipio, PR\"\t72023\t\"San Germ?n Municipio, PR\"\t72125\n\"Caguas Municipio, PR\"\t72025\t\"Aguas Buenas Municipio, PR\"\t72007\n\"Caguas Municipio, PR\"\t72025\t\"Caguas Municipio, PR\"\t72025\n\"Caguas Municipio, PR\"\t72025\t\"Cayey Municipio, PR\"\t72035\n\"Caguas Municipio, PR\"\t72025\t\"Cidra Municipio, PR\"\t72041\n\"Caguas Municipio, PR\"\t72025\t\"Gurabo Municipio, PR\"\t72063\n\"Caguas Municipio, PR\"\t72025\t\"San Juan Municipio, PR\"\t72127\n\"Caguas Municipio, PR\"\t72025\t\"San Lorenzo Municipio, PR\"\t72129\n\"Caguas Municipio, PR\"\t72025\t\"Trujillo Alto Municipio, PR\"\t72139\n\"Camuy Municipio, PR\"\t72027\t\"Camuy Municipio, PR\"\t72027\n\"Camuy Municipio, PR\"\t72027\t\"Hatillo Municipio, PR\"\t72065\n\"Camuy Municipio, PR\"\t72027\t\"Lares Municipio, PR\"\t72081\n\"Camuy Municipio, PR\"\t72027\t\"Quebradillas Municipio, PR\"\t72115\n\"Camuy Municipio, PR\"\t72027\t\"San Sebasti?n Municipio, PR\"\t72131\n\"Can?vanas Municipio, PR\"\t72029\t\"Can?vanas Municipio, PR\"\t72029\n\"Can?vanas Municipio, PR\"\t72029\t\"Carolina Municipio, PR\"\t72031\n\"Can?vanas Municipio, PR\"\t72029\t\"Gurabo Municipio, PR\"\t72063\n\"Can?vanas Municipio, PR\"\t72029\t\"Juncos Municipio, PR\"\t72077\n\"Can?vanas Municipio, PR\"\t72029\t\"Las Piedras Municipio, PR\"\t72085\n\"Can?vanas Municipio, PR\"\t72029\t\"Lo?za Municipio, PR\"\t72087\n\"Can?vanas Municipio, PR\"\t72029\t\"R?o Grande Municipio, PR\"\t72119\n\"Carolina Municipio, PR\"\t72031\t\"Can?vanas Municipio, PR\"\t72029\n\"Carolina Municipio, PR\"\t72031\t\"Carolina Municipio, PR\"\t72031\n\"Carolina Municipio, PR\"\t72031\t\"Gurabo Municipio, PR\"\t72063\n\"Carolina Municipio, PR\"\t72031\t\"Juncos Municipio, PR\"\t72077\n\"Carolina Municipio, PR\"\t72031\t\"Lo?za Municipio, PR\"\t72087\n\"Carolina Municipio, PR\"\t72031\t\"San Juan Municipio, PR\"\t72127\n\"Carolina Municipio, PR\"\t72031\t\"Trujillo Alto Municipio, PR\"\t72139\n\"Cata?o Municipio, PR\"\t72033\t\"Bayam?n Municipio, PR\"\t72021\n\"Cata?o Municipio, PR\"\t72033\t\"Cata?o Municipio, PR\"\t72033\n\"Cata?o Municipio, PR\"\t72033\t\"Guaynabo Municipio, PR\"\t72061\n\"Cata?o Municipio, PR\"\t72033\t\"San Juan Municipio, PR\"\t72127\n\"Cata?o Municipio, PR\"\t72033\t\"Toa Baja Municipio, PR\"\t72137\n\"Cayey Municipio, PR\"\t72035\t\"Aibonito Municipio, PR\"\t72009\n\"Cayey Municipio, PR\"\t72035\t\"Caguas Municipio, PR\"\t72025\n\"Cayey Municipio, PR\"\t72035\t\"Cayey Municipio, PR\"\t72035\n\"Cayey Municipio, PR\"\t72035\t\"Cidra Municipio, PR\"\t72041\n\"Cayey Municipio, PR\"\t72035\t\"Guayama Municipio, PR\"\t72057\n\"Cayey Municipio, PR\"\t72035\t\"Patillas Municipio, PR\"\t72109\n\"Cayey Municipio, PR\"\t72035\t\"Salinas Municipio, PR\"\t72123\n\"Cayey Municipio, PR\"\t72035\t\"San Lorenzo Municipio, PR\"\t72129\n\"Ceiba Municipio, PR\"\t72037\t\"Ceiba Municipio, PR\"\t72037\n\"Ceiba Municipio, PR\"\t72037\t\"Culebra Municipio, PR\"\t72049\n\"Ceiba Municipio, PR\"\t72037\t\"Fajardo Municipio, PR\"\t72053\n\"Ceiba Municipio, PR\"\t72037\t\"Luquillo Municipio, PR\"\t72089\n\"Ceiba Municipio, PR\"\t72037\t\"Naguabo Municipio, PR\"\t72103\n\"Ceiba Municipio, PR\"\t72037\t\"R?o Grande Municipio, PR\"\t72119\n\"Ceiba Municipio, PR\"\t72037\t\"Vieques Municipio, PR\"\t72147\n\"Ciales Municipio, PR\"\t72039\t\"Arecibo Municipio, PR\"\t72013\n\"Ciales Municipio, PR\"\t72039\t\"Ciales Municipio, PR\"\t72039\n\"Ciales Municipio, PR\"\t72039\t\"Florida Municipio, PR\"\t72054\n\"Ciales Municipio, PR\"\t72039\t\"Jayuya Municipio, PR\"\t72073\n\"Ciales Municipio, PR\"\t72039\t\"Manat? Municipio, PR\"\t72091\n\"Ciales Municipio, PR\"\t72039\t\"Morovis Municipio, PR\"\t72101\n\"Ciales Municipio, PR\"\t72039\t\"Orocovis Municipio, PR\"\t72107\n\"Ciales Municipio, PR\"\t72039\t\"Utuado Municipio, PR\"\t72141\n\"Cidra Municipio, PR\"\t72041\t\"Aguas Buenas Municipio, PR\"\t72007\n\"Cidra Municipio, PR\"\t72041\t\"Aibonito Municipio, PR\"\t72009\n\"Cidra Municipio, PR\"\t72041\t\"Barranquitas Municipio, PR\"\t72019\n\"Cidra Municipio, PR\"\t72041\t\"Caguas Municipio, PR\"\t72025\n\"Cidra Municipio, PR\"\t72041\t\"Cayey Municipio, PR\"\t72035\n\"Cidra Municipio, PR\"\t72041\t\"Cidra Municipio, PR\"\t72041\n\"Cidra Municipio, PR\"\t72041\t\"Comer?o Municipio, PR\"\t72045\n\"Coamo Municipio, PR\"\t72043\t\"Aibonito Municipio, PR\"\t72009\n\"Coamo Municipio, PR\"\t72043\t\"Barranquitas Municipio, PR\"\t72019\n\"Coamo Municipio, PR\"\t72043\t\"Coamo Municipio, PR\"\t72043\n\"Coamo Municipio, PR\"\t72043\t\"Juana D?az Municipio, PR\"\t72075\n\"Coamo Municipio, PR\"\t72043\t\"Orocovis Municipio, PR\"\t72107\n\"Coamo Municipio, PR\"\t72043\t\"Salinas Municipio, PR\"\t72123\n\"Coamo Municipio, PR\"\t72043\t\"Santa Isabel Municipio, PR\"\t72133\n\"Coamo Municipio, PR\"\t72043\t\"Villalba Municipio, PR\"\t72149\n\"Comer?o Municipio, PR\"\t72045\t\"Aguas Buenas Municipio, PR\"\t72007\n\"Comer?o Municipio, PR\"\t72045\t\"Barranquitas Municipio, PR\"\t72019\n\"Comer?o Municipio, PR\"\t72045\t\"Bayam?n Municipio, PR\"\t72021\n\"Comer?o Municipio, PR\"\t72045\t\"Cidra Municipio, PR\"\t72041\n\"Comer?o Municipio, PR\"\t72045\t\"Comer?o Municipio, PR\"\t72045\n\"Comer?o Municipio, PR\"\t72045\t\"Naranjito Municipio, PR\"\t72105\n\"Corozal Municipio, PR\"\t72047\t\"Barranquitas Municipio, PR\"\t72019\n\"Corozal Municipio, PR\"\t72047\t\"Corozal Municipio, PR\"\t72047\n\"Corozal Municipio, PR\"\t72047\t\"Morovis Municipio, PR\"\t72101\n\"Corozal Municipio, PR\"\t72047\t\"Naranjito Municipio, PR\"\t72105\n\"Corozal Municipio, PR\"\t72047\t\"Orocovis Municipio, PR\"\t72107\n\"Corozal Municipio, PR\"\t72047\t\"Toa Alta Municipio, PR\"\t72135\n\"Corozal Municipio, PR\"\t72047\t\"Vega Alta Municipio, PR\"\t72143\n\"Culebra Municipio, PR\"\t72049\t\"Ceiba Municipio, PR\"\t72037\n\"Culebra Municipio, PR\"\t72049\t\"Culebra Municipio, PR\"\t72049\n\"Dorado Municipio, PR\"\t72051\t\"Dorado Municipio, PR\"\t72051\n\"Dorado Municipio, PR\"\t72051\t\"Toa Alta Municipio, PR\"\t72135\n\"Dorado Municipio, PR\"\t72051\t\"Toa Baja Municipio, PR\"\t72137\n\"Dorado Municipio, PR\"\t72051\t\"Vega Alta Municipio, PR\"\t72143\n\"Fajardo Municipio, PR\"\t72053\t\"Ceiba Municipio, PR\"\t72037\n\"Fajardo Municipio, PR\"\t72053\t\"Fajardo Municipio, PR\"\t72053\n\"Fajardo Municipio, PR\"\t72053\t\"Luquillo Municipio, PR\"\t72089\n\"Florida Municipio, PR\"\t72054\t\"Arecibo Municipio, PR\"\t72013\n\"Florida Municipio, PR\"\t72054\t\"Barceloneta Municipio, PR\"\t72017\n\"Florida Municipio, PR\"\t72054\t\"Ciales Municipio, PR\"\t72039\n\"Florida Municipio, PR\"\t72054\t\"Florida Municipio, PR\"\t72054\n\"Florida Municipio, PR\"\t72054\t\"Manat? Municipio, PR\"\t72091\n\"Gu?nica Municipio, PR\"\t72055\t\"Gu?nica Municipio, PR\"\t72055\n\"Gu?nica Municipio, PR\"\t72055\t\"Guayanilla Municipio, PR\"\t72059\n\"Gu?nica Municipio, PR\"\t72055\t\"Lajas Municipio, PR\"\t72079\n\"Gu?nica Municipio, PR\"\t72055\t\"Sabana Grande Municipio, PR\"\t72121\n\"Gu?nica Municipio, PR\"\t72055\t\"Yauco Municipio, PR\"\t72153\n\"Guayama Municipio, PR\"\t72057\t\"Arroyo Municipio, PR\"\t72015\n\"Guayama Municipio, PR\"\t72057\t\"Cayey Municipio, PR\"\t72035\n\"Guayama Municipio, PR\"\t72057\t\"Guayama Municipio, PR\"\t72057\n\"Guayama Municipio, PR\"\t72057\t\"Patillas Municipio, PR\"\t72109\n\"Guayama Municipio, PR\"\t72057\t\"Salinas Municipio, PR\"\t72123\n\"Guayanilla Municipio, PR\"\t72059\t\"Adjuntas Municipio, PR\"\t72001\n\"Guayanilla Municipio, PR\"\t72059\t\"Gu?nica Municipio, PR\"\t72055\n\"Guayanilla Municipio, PR\"\t72059\t\"Guayanilla Municipio, PR\"\t72059\n\"Guayanilla Municipio, PR\"\t72059\t\"Pe?uelas Municipio, PR\"\t72111\n\"Guayanilla Municipio, PR\"\t72059\t\"Yauco Municipio, PR\"\t72153\n\"Guaynabo Municipio, PR\"\t72061\t\"Aguas Buenas Municipio, PR\"\t72007\n\"Guaynabo Municipio, PR\"\t72061\t\"Bayam?n Municipio, PR\"\t72021\n\"Guaynabo Municipio, PR\"\t72061\t\"Cata?o Municipio, PR\"\t72033\n\"Guaynabo Municipio, PR\"\t72061\t\"Guaynabo Municipio, PR\"\t72061\n\"Guaynabo Municipio, PR\"\t72061\t\"San Juan Municipio, PR\"\t72127\n\"Gurabo Municipio, PR\"\t72063\t\"Caguas Municipio, PR\"\t72025\n\"Gurabo Municipio, PR\"\t72063\t\"Can?vanas Municipio, PR\"\t72029\n\"Gurabo Municipio, PR\"\t72063\t\"Carolina Municipio, PR\"\t72031\n\"Gurabo Municipio, PR\"\t72063\t\"Gurabo Municipio, PR\"\t72063\n\"Gurabo Municipio, PR\"\t72063\t\"Juncos Municipio, PR\"\t72077\n\"Gurabo Municipio, PR\"\t72063\t\"San Lorenzo Municipio, PR\"\t72129\n\"Gurabo Municipio, PR\"\t72063\t\"Trujillo Alto Municipio, PR\"\t72139\n\"Hatillo Municipio, PR\"\t72065\t\"Arecibo 
